vi "Enbl-Dsbl-Ctrl's.vi"(0 "Quick-GUI-Update in":refnum<class "Quick-GUI-Update.lvclass">, 2 "Ctrl-Label":string[](array[string]), 11 "error in (no error)":errorcluster, 13 "Enbl-Dsbl":i32=3) -> (4 "Quick-GUI-Update out":refnum<class "Quick-GUI-Update.lvclass">, 15 "error out":errorcluster)   [LabVIEW 2020, in "Easy GUI Operation.lvlib" / "Quick-GUI-Update.lvclass"]
doc: "<b>Enable Disable</b>\n1---><b>Enable</b> control's based on the Ctrl-Label input.\n2---><b>Disable</b> control's based on the Ctrl-Label input.\n3---><b>Diable and Grayed Out</b> control's based on the Ctrl-Label input.\n4---><b>Enable All</b> control's present in the front panel."
uses:
  Quick-GUI-Update.lvclass
  Quick-GUI-Update.lvclass/Quick-GUI-Update.ctl
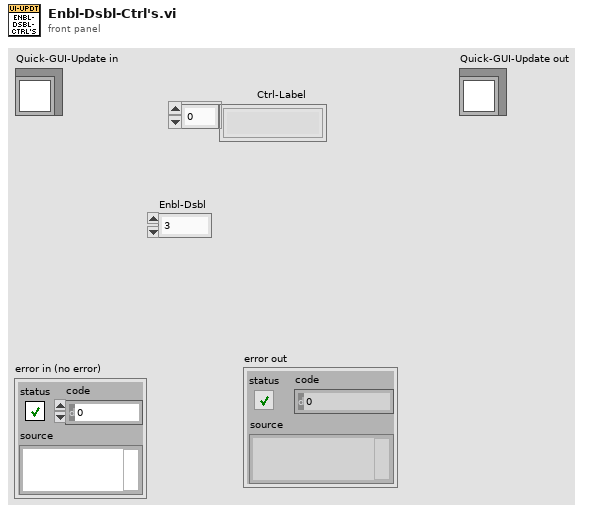
[diagram p1: front panel]
types:
  T1 = map{string, set{cluster{"Ctrl-Ref":refnum<vi>, "Ctrl Index":i32, "Class-Name":string, "Class ID":u32}}}
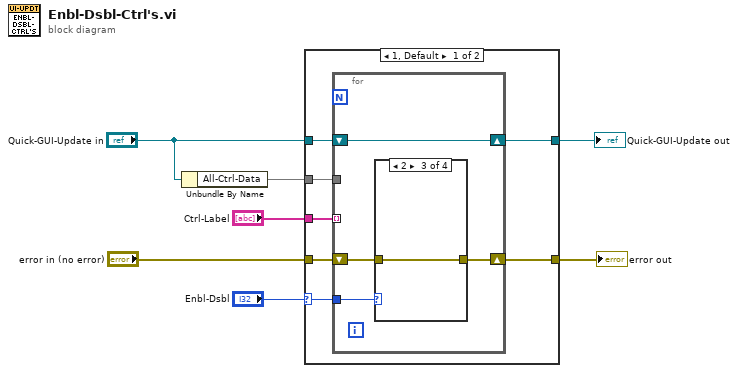
[diagram p0: block diagram]
diagram:
  n1 = Unbundle By Name("Quick-GUI-Update in") -> ("All-Ctrl-Data"=w3:T1)
  n2 = case shown="1, Default" "Enbl-Dsbl" {
    selector: "Enbl-Dsbl" -> [w8 _]
    tunnel: "Ctrl-Label" -> [w14 _]
    tunnel: w3 -> [w13 w27]
    tunnel: "error in (no error)" -> [w12 w26]
    tunnel: "Quick-GUI-Update in" -> [w11 w25]
    tunnel: [w10 w24] -> w6
    tunnel: [w9 w23] -> w5
    frame 1, Default {
      n3 = for {
        tunnel: w14 -> [_] mode=indexing
        tunnel: w13 -> [_]
        tunnel: w8 -> [w17]
        shift-right: [w18] -> w9
        shift-left: w12 -> [w15]
        shift-right: [w16] -> w10
        shift-left: w11 -> [w16]
        n4 = case shown="2" w17 {
          tunnel: w15 -> [w19 w20 w21 w22]
          tunnel: [w19 w20 w21 w22] -> w18
          frame 0, Default {
          }
          frame 1 {
          }
          frame 2 {
          }
          frame 3 {
          }
        }
      }
    }
    frame 4 {
      n5 = for {
        tunnel: w27 -> [_] mode=indexing
        shift-right: [w28] -> w23
        shift-left: w26 -> [w28]
        shift-right: [w29] -> w24
        shift-left: w25 -> [w29]
      }
    }
  }
  "Quick-GUI-Update out" <- w6
  "error out" <- w5
